vi "Get AI param from PGserver sh1.vi"(6 "conninfo":T2={"host"="localhost", "port"="5432", "client_encoding"="WIN1251", "dbname"="data", "user"="postgres", "password"=""}, 8 "error in (no error)":errorcluster, 9 "AIParamColumns":string[](array[string])=["instrument_gain", "instrument_offset", "time_const", "instrument_min_offset", "instrument_range_min", "process_range_min", "process_low_acd", "process_low_alr", "process_high_alr", "process_high_acd", "process_range_max", "instrument_range_max", "instrument_max_offset", "d", "input_register_min", "input_register_max", "input_pv_min", "input_pv_max", "fcode", "fcodef", "fcode_full", "fname", "process_units"], 10 "AIParamTable":string="fa_3", 11 "AIParameters":string[](array[string])) -> (0 "error out":errorcluster, 2 "Names table":string[][](array[string]), 3 "Parameters table":dbl[][](array[numeric]))   [LabVIEW 2019, in "Inputs.lvlib"]
uses:
  Inputs.lvlib
  Database/ctl/Coninfo.ctl
  Database/PostgreSQL2LabVIEW/libpqlv/src/PQfinish.vi
  Database/PostgreSQL2LabVIEW/libpqlv/src/PQconnectdb.vi
  Database/PostgreSQL2LabVIEW/libpqlv/src/PQerrorMessage.vi
  Database/PostgreSQL2LabVIEW/libpqlv/src/PQstatus.vi
  <vilib>/dlg_ctls.llb/Space Constant.vi
  Database/Progress.vi
  Database/PostgreSQL.lvlib
  Database/PostgreSQL2LabVIEW/libpqUtility64/libpqutility64.lvlib
  Database/PostgreSQL2LabVIEW/libpqUtility/libpqutility.lvlib
panel:
  out "PQStatus":T1(ring)
  # "fcode_full"
  # "fname"
  # "process_unit"
  # "time_const"
  # "instrument_min_offset"
  # "process_range_min"
  # "process_low_acd"
  # "instrument_range_max"
  # "d"
  # "input_register_min"
  # "input_register_max"
  # "input_pv_min"
  # "input_pv_max"
  # "fcodef"
  # "instrument_max_offset"
  # "instrument_range_min"
  # "process_range_max"
  # "instrument_offset"
  # "process_high_acd"
  # "process_high_alr"
  # "instrument_gain"
  # "process_low_alr"
  # "fcode"
  # "Names"
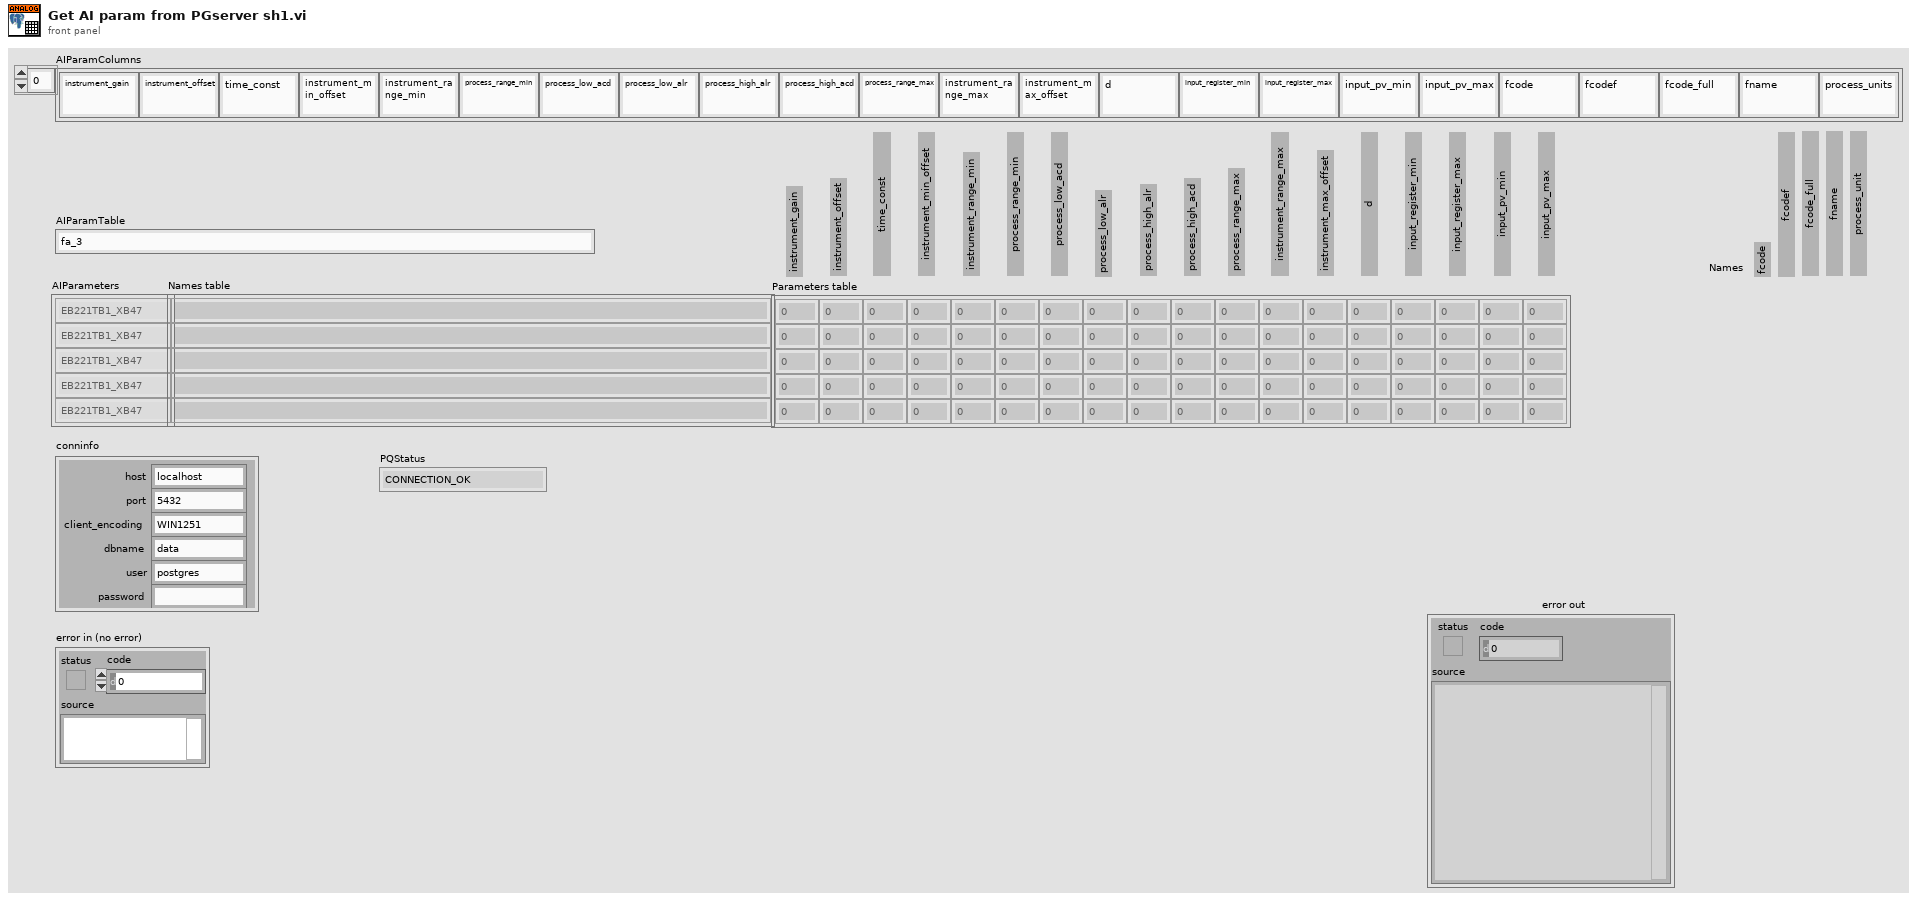
[diagram p1: front panel]
types:
  T1 = enum32{"CONNECTION_OK", "CONNECTION_BAD", "CONNECTION_STARTED", "CONNECTION_MADE", "CONNECTION_AWAITING_RESPONSE", "CONNECTION_AUTH_OK", "CONNECTION_SETENV", "CONNECTION_SSL_STARTUP", "CONNECTION_NEEDED"}
  T2 = typedef "PostgreSQL.lvlib/Coninfo.ctl" = cluster{"host":string, "port":string, "client_encoding":string, "dbname":string, "user":string, "password":string}
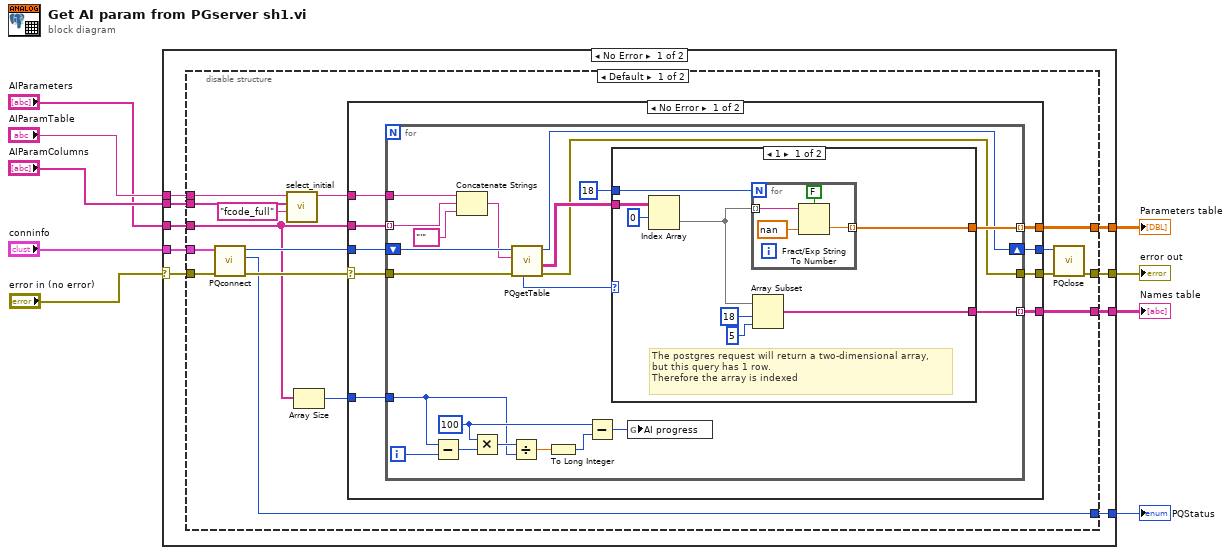
[diagram p0: block diagram]
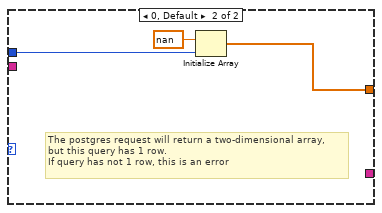
[diagram p2: hidden frame]
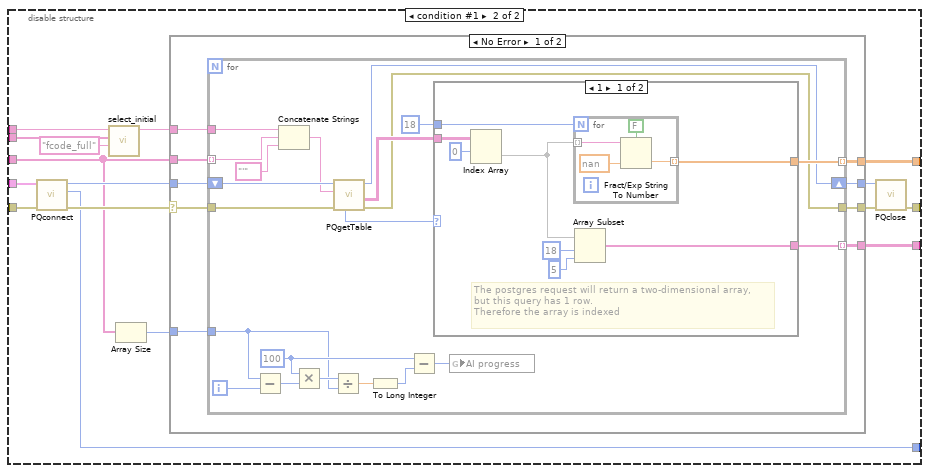
[diagram p4: hidden frame]
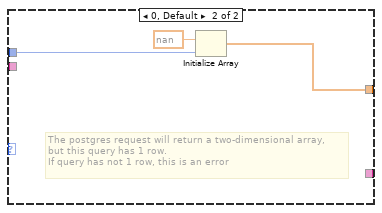
[diagram p5: hidden frame]
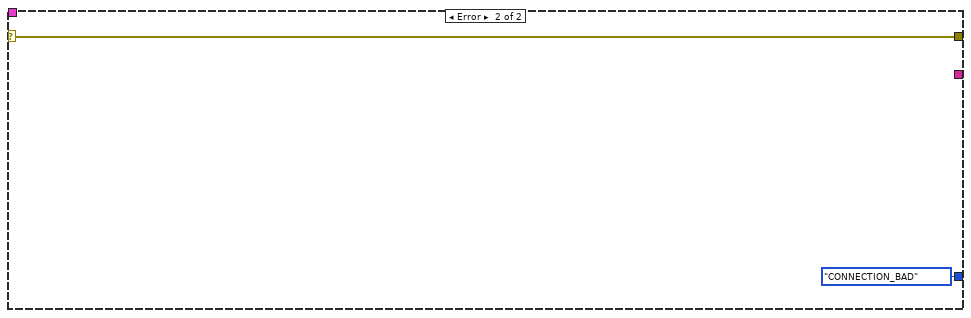
[diagram p7: hidden frame]
diagram:
  n1 = case shown="No Error" "error in (no error)" {
    selector: "error in (no error)" -> [w11 w146]
    tunnel: [w18 w146] -> w9
    tunnel: [w17 _] -> w8
    tunnel: [w16 _] -> w7
    tunnel: "AIParamColumns" -> [w15 _]
    tunnel: "conninfo" -> [w14 _]
    tunnel: "AIParamTable" -> [w13 _]
    tunnel: "AIParameters" -> [w12 _]
    tunnel: [w10 T1."CONNECTION_BAD" ("PQStatus")] -> w1
    frame No Error {
      n2 = disable-structure shown="Default" {
        disable-tunnel: [w19 w83] -> w18
        disable-tunnel: [w24 w94] -> w17
        disable-tunnel: [w23 w89] -> w16
        disable-tunnel: w15 -> [w26 w92]
        disable-tunnel: w14 -> [w29 w91]
        disable-tunnel: w13 -> [w27 w93]
        disable-tunnel: w12 -> [w25 w95]
        disable-tunnel: w11 -> [w28 w90]
        disable-tunnel: [w22 w85] -> w10
        frame condition #0 (active) {
          n3 = call "PQconnect.vi"("error in (no error)"=w28, "conninfo"=w29) -> ("error out"=w34:errorcluster, "PQStatus"=w22:T1, "conn"=w33:u32)  [unwired: 7 in]
          n4 = call "select_initial.vi"("Column name"="fcode_full", "Column table"=w26, "table"=w27) -> ("parameters"=w31:string)  [unwired: 7 in, 1 out]
          n5 = Array Size(array=w25) -> (size(s)=w32:i32)
          n6 = case shown="No Error" w34 {
            selector: w34 -> [w41 w81]
            tunnel: w25 -> [w39 _]
            tunnel: [w43 _] -> w24
            tunnel: [w42 _] -> w23
            tunnel: w32 -> [w40 _]
            tunnel: w33 -> [w38 w80]
            tunnel: w31 -> [w37 _]
            tunnel: [w36 w81] -> w20
            tunnel: [w35 w80] -> w21
            frame No Error {
              n7 = for {
                tunnel: [w64] -> w42 mode=indexing
                tunnel: [w63] -> w43 mode=indexing
                tunnel: w41 -> [w50]
                tunnel: w40 -> [w53]
                tunnel: w39 -> [w52] mode=indexing
                tunnel: w37 -> [w62]
                tunnel: [w45] -> w36
                shift-right: [w44] -> w35
                shift-left: w38 -> [w51]
                i -> [w54]
                w58 = 100 ("y")
                n8 = Subtract(x=w53, y=w54) -> (x-y=w57:i32)
                n9 = Concatenate Strings(w62, w52, "'" ("table")) -> (w49:string)
                n10 = Multiply(x=w58, y=w57) -> (x*y=w60:i32)
                n11 = Divide(x=w60, y=w53) -> (x/y=w56:dbl)
                n12 = call "PQgetTable.vi"("error in"=w50, "query"=w49, "conn"=w51) -> ("error out"=w45:errorcluster, "Data"=w48:string[][], "conn_out"=w44:u32, "PQnTuples"=w47:i32)  [unwired: 4 in, 1 out]
                n13 = To Long Integer(number=w56) -> (32bit integer=w55:i32)
                n14 = Subtract(x=w58, y=w55) -> (x-y=w59:i32)
                n15 = case shown="1" w47 {
                  tunnel: [w65 w78] -> w63
                  tunnel: 18 ("y") -> [w68 w77]
                  tunnel: w48 -> [w67 _]
                  tunnel: [w70 _] -> w64
                  frame 1 {
                    # "The postgres request will return a two-dimensional array,\nbut this query has 1 row.\nTherefore the array is indexed"
                    n16 = Index Array(array=w67, index (row)=0) -> (element=w66:string[])  [unwired: 1 in]
                    n17 = for {
                      N: w68 -> [_]
                      tunnel: w66 -> [w75] mode=indexing
                      tunnel: [w74] -> w65 mode=indexing
                      n18 = Fract/Exp String To Number(use system decimal point (T)=FALSE, string=w75, default (0 dbl)=nan) -> (number=w74:dbl)  [unwired: 1 in, 1 out]
                    }
                    n19 = Array Subset(array=w66, index=18, length=5) -> (w70:string[])
                  }
                  frame 0, Default {
                    # "The postgres request will return a two-dimensional array,\nbut this query has 1 row.\nIf query has not 1 row, this is an error"
                    n20 = Initialize Array(nan, w77) -> (w78:dbl[])
                  }
                }
                n21 = global write "Progress.vi" "AI progress"(w59) -> ()
              }
            }
            frame Error {
            }
          }
          n22 = call "PQclose.vi"("error in (no error)"=w20, "conn"=w21) -> ("error out"=w19:errorcluster)  [unwired: 9 in]
        }
        frame condition #1 {
          n23 = call "PQconnect.vi"("error in (no error)"=w90, "conninfo"=w91) -> ("error out"=w97:errorcluster, "PQStatus"=w85:T1, "conn"=w96:u64)  [unwired: 7 in]
          n24 = call "select_initial.vi"("Column name"="fcode_full", "Column table"=w92, "table"=w93) -> ("parameters"=w87:string)  [unwired: 7 in, 1 out]
          n25 = Array Size(array=w95) -> (size(s)=w88:i32)
          n26 = case shown="No Error" w97 {
            selector: w97 -> [w104 w143]
            tunnel: w95 -> [w102 _]
            tunnel: [w106 _] -> w94
            tunnel: [w105 _] -> w89
            tunnel: w88 -> [w103 _]
            tunnel: w96 -> [w101 w144]
            tunnel: w87 -> [w100 _]
            tunnel: [w99 w143] -> w82
            tunnel: [w98 w144] -> w84
            frame No Error {
              n27 = for {
                tunnel: [w127] -> w105 mode=indexing
                tunnel: [w126] -> w106 mode=indexing
                tunnel: w104 -> [w113]
                tunnel: w103 -> [w116]
                tunnel: w102 -> [w115] mode=indexing
                tunnel: w100 -> [w125]
                tunnel: [w108] -> w99
                shift-right: [w107] -> w98
                shift-left: w101 -> [w114]
                i -> [w117]
                w121 = 100 ("y")
                n28 = Subtract(x=w116, y=w117) -> (x-y=w120:i32)
                n29 = Concatenate Strings(w125, w115, "'" ("table")) -> (w112:string)
                n30 = Multiply(x=w121, y=w120) -> (x*y=w123:i32)
                n31 = Divide(x=w123, y=w116) -> (x/y=w119:dbl)
                n32 = call "PQgetTable.vi"("error in"=w113, "query"=w112, "conn"=w114) -> ("error out"=w108:errorcluster, "Data"=w111:string[][], "conn_out"=w107:u64, "PQnTuples"=w110:i64)  [unwired: 4 in, 1 out]
                n33 = To Long Integer(number=w119) -> (32bit integer=w118:i32)
                n34 = Subtract(x=w121, y=w118) -> (x-y=w122:i32)
                n35 = case shown="1" w110 {
                  tunnel: [w128 w141] -> w126
                  tunnel: 18 ("y") -> [w131 w140]
                  tunnel: w111 -> [w130 _]
                  tunnel: [w133 _] -> w127
                  frame 1 {
                    # "The postgres request will return a two-dimensional array,\nbut this query has 1 row.\nTherefore the array is indexed"
                    n36 = Index Array(array=w130, index (row)=0) -> (element=w129:string[])  [unwired: 1 in]
                    n37 = for {
                      N: w131 -> [_]
                      tunnel: w129 -> [w138] mode=indexing
                      tunnel: [w137] -> w128 mode=indexing
                      n38 = Fract/Exp String To Number(use system decimal point (T)=FALSE, string=w138, default (0 dbl)=nan) -> (number=w137:dbl)  [unwired: 1 in, 1 out]
                    }
                    n39 = Array Subset(array=w129, index=18, length=5) -> (w133:string[])
                  }
                  frame 0, Default {
                    # "The postgres request will return a two-dimensional array,\nbut this query has 1 row.\nIf query has not 1 row, this is an error"
                    n40 = Initialize Array(nan, w140) -> (w141:dbl[])
                  }
                }
                n41 = global write "Progress.vi" "AI progress"(w122) -> ()
              }
            }
            frame Error {
            }
          }
          n42 = call "PQclose.vi"("error in (no error)"=w82, "conn"=w84) -> ("error out"=w83:errorcluster)  [unwired: 9 in]
        }
      }
    }
    frame Error {
    }
  }
  "error out" <- w9
  "Parameters table" <- w8
  "Names table" <- w7
  "PQStatus" <- w1
